vi "GetErrCodes.vi"(0 "Error":u16(ring)=2 items=["TopicReadTimeout", "Read=SS", "GetQueueErr", "NoMaster", "Write=PS", "Unparse", "ServiceReply"], 1 "Added Textt":string, 2 "Supported Errors":string[](array[string])=["TopicReadTimeout", "Read=SS", "GetQueueErr", "NoMaster", "Write=PS", "Unparse", "ServiceReply"], 4 "Errors":errorcluster[](array[cluster])=[{"status"=FALSE, "code"=1, "source"="Topic read timeout"}, {"status"=TRUE, "code"=2, "source"="Can only read a subscriber or service"}, {"status"=TRUE, "code"=4, "source"="Error in finding queue"}, {"status"=TRUE, "code"=5, "source"="No Master Found"}, {"status"=TRUE, "code"=3, "source"="Can only write to a publisher or service"}, {"status"=FALSE, "code"=74, "source"="Error in parsing a %s"}, {"status"=TRUE, "code"=6, "source"="Service reply error (%s)"}]) -> (3 "Error":errorcluster={"status"=TRUE, "code"=4, "source"="Error in finding queue"})   [LabVIEW 2012]
uses:
  <vilib>/ErrorRing/Error Ring.xnode
panel:
  in  "REGrab":bool
  out "text":string="TopicReadTimeout(1)W Topic read timeout\nRead=SS(2)E Can only read a subscriber or service\nGetQueueErr(4)E Error in finding queue\nNoMaster(5)E No Master Found\nWrite=PS(3)E Can only write to a publisher or service\nUnparse(74)W Error in parsing a %s\nServiceReply(6)E Service reply error (%s)\n"
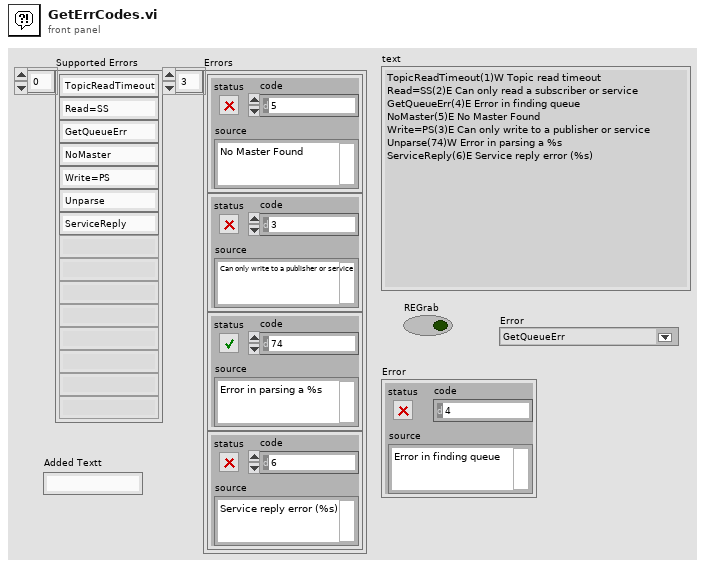
[diagram p1: front panel]
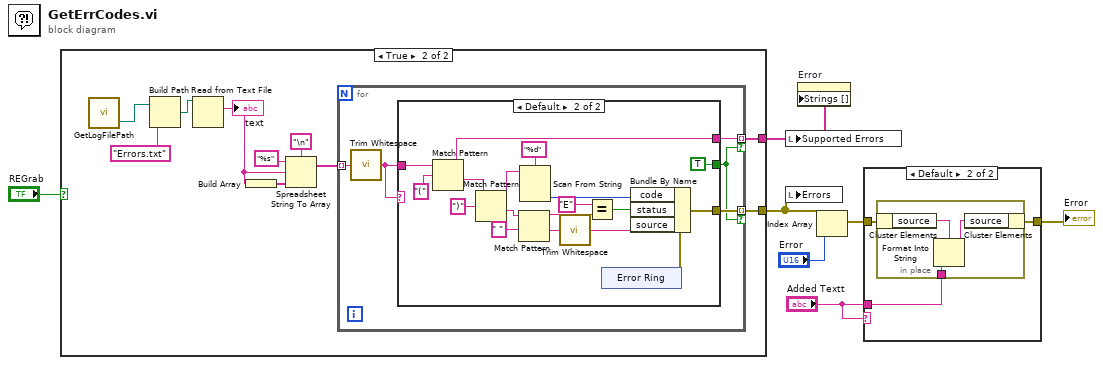
[diagram p0: block diagram]
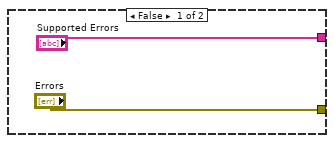
[diagram p2: hidden frame]
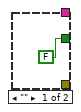
[diagram p3: hidden frame]
diagram:
  n1 = case shown="True" "REGrab" {
    tunnel: ["Errors" w11] -> w2
    tunnel: ["Supported Errors" w10] -> w1
    frame False {
    }
    frame True {
      n2 = call <userlib>:"GetLogFilePath.vi"() -> ("LogFolder"=w17:path)  [unwired: 2 in, 1 out]
      n3 = Build Path(base path=w17, name or relative path="Errors.txt" ("Server name")) -> (appended path=w19:path)
      n4 = Read from Text File(file (use dialog)=w19) -> (text=w14:string)  [unwired: 3 in, 3 out]
      "text" <- w14
      n5 = Build Array(w14) -> (w13:string[])
      n6 = Spreadsheet String To Array(delimiter (Tab)="\n", format string="%s", spreadsheet string=w14, array type (2D Dbl)=w13) -> (array=w12:string[])
      n7 = for {
        tunnel: w12 -> [w24] mode=indexing
        tunnel: [w20] -> w10 mode=indexing if=w21
        tunnel: [w23] -> w11 mode=indexing if=w21
        n8 = call <vilib>:"Trim Whitespace.vi"("string"=w24) -> ("trimmed string"=w22:string)  [unwired: 1 in]
        n9 = case shown="Default" w22 {
          tunnel: w22 -> [_ w43]
          tunnel: [_ w36] -> w20
          tunnel: [_ w27] -> w23
          tunnel: [FALSE TRUE] -> w21
          frame "" {
          }
          frame Default {
            n10 = Match Pattern(string=w43, regular expression="(") -> (before substring=w36:string, after substring=w40:string)  [unwired: 1 in, 2 out]
            n11 = Match Pattern(string=w40, regular expression=")") -> (before substring=w35:string, after substring=w39:string)  [unwired: 1 in, 2 out]
            n12 = Match Pattern(string=w39, regular expression=" ") -> (before substring=w33:string, after substring=w37:string)  [unwired: 1 in, 2 out]
            n13 = Scan From String(format string="%d", input string=w35) -> (output 1=w28:i32)  [unwired: 3 in, 3 out]
            n14 = call <vilib>:"Trim Whitespace.vi"("string"=w37) -> ("trimmed string"=w31:string)  [unwired: 1 in]
            n15 = Equal?(x="E", y=w33) -> (x = y?=w29:bool)
            n16 = xnode "Error Ring"() -> ("error out"=w32:errorcluster)
            n17 = Bundle By Name(cluster=w32, "code"=w28, "status"=w29, "source"=w31) -> (w27:errorcluster)
          }
        }
      }
    }
  }
  n18 = local write "Supported Errors"(w1) -> ()
  n19 = local write "Errors"(w2) -> ()
  n20 = property on="Error" class="Ring (strict)"("Strings []"=w1) -> ()  [unwired: 2 in, 2 out]
  n21 = Index Array(array=w2, index="Error") -> (element=w6:errorcluster)
  n22 = case shown="Default" "Added Textt" {
    tunnel: w6 -> [w45 w48]
    tunnel: [w45 w47] -> w5
    tunnel: "Added Textt" -> [_ w46]
    frame "" {
    }
    frame Default {
      n23 = in-place {
        in-place-border: w46 -> [w49]
        n24 = in-place-cluster #1(w48) -> ("source"=w51:string)
        n25 = Format Into String(format string=w51, w49) -> (resulting string=w50:string)  [unwired: 2 in, 1 out]
        n26 = in-place-cluster #1("source"=w50) -> (w47:errorcluster)
      }
    }
  }
  "Error" <- w5
